vi "模板读取.vi"(1 "Path":path) -> (0 "模板特征参数":dbl[][](array[numeric]))   [LabVIEW 2018]
panel:
  out "Filename Out":path caption="文件名输出"
  out "模板特征参数 2":dbl[][](array[numeric])
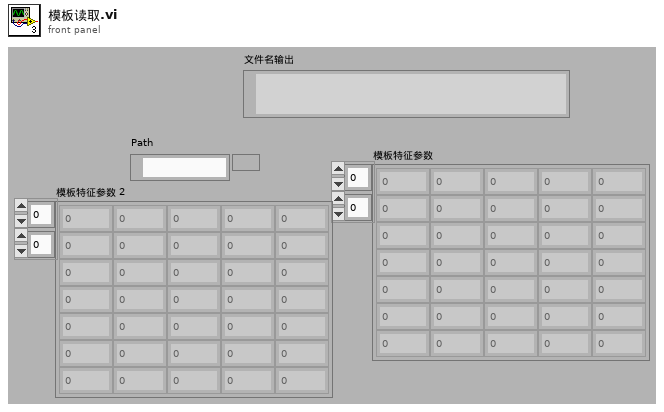
[diagram p1: front panel]
types:
  T1 = enum16{"open", "replace", "create", "open or create", "replace or create", "replace or create with confirmation"}
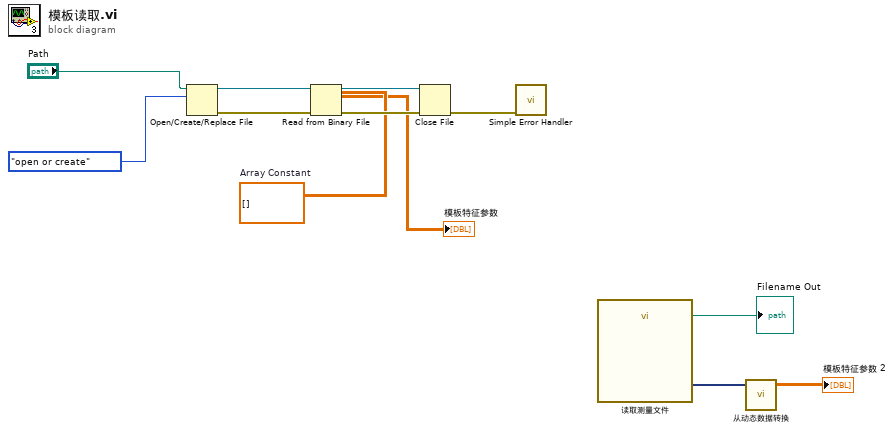
[diagram p0: block diagram]
diagram:
  w5 = dbl[][] []  # Array Constant
  n1 = Open/Create/Replace File(file path (use dialog)="Path", operation (0:open)=T1."open or create") -> (refnum out=w9:refnum<file>, error out=w10:errorcluster)  [unwired: 4 in, 1 out]
  n2 = Read from Binary File(5:w5, 8:w10, 11:w9) -> (0:w12:errorcluster, 2:→"模板特征参数":dbl[][], 3:w7:refnum<file>)  [unwired: 3 in, 1 out]
  n3 = Close File(refnum=w7, error in=w12) -> (error out=w11:errorcluster)  [unwired: 1 out]
  n4 = call <vilib>:"Simple Error Handler.vi"("error in (no error)"=w11) -> ()  [unwired: 4 in, 5 out]
  n5 = call "读取测量文件"() -> ("Filename Out"=→"Filename Out":path, "Signals"=w3:dynamicdata)  [unwired: 6 in, 4 out]
  n6 = call "从动态数据转换"("Dynamic Data Type"=w3) -> ("Array"=→"模板特征参数 2":dbl[][])  [unwired: 3 in]
